vi "Find Parameter by Name.vi"(8 "error in":errorcluster, 10 "parameter name":string, 11 "label ref":T1 format="%.0x") -> (0 "error out":errorcluster, 2 "parameter ref":T1 format="%.0x", 3 "label ref out":T1 format="%.0x", 4 "found?":bool)   [LabVIEW 2024, in "AIM ARINC 429 Scripting.lvlib"]
doc: "Within the specified <b>label ref</b>, this VI searches for a parameter with matching <b>parameter name</b>. If a match is found, returns the matching <b>parameter</b> reference. If no match is found, the returned reference is invalid and <b>found?</b> equals False."
uses:
  AIM ARINC 429 Scripting.lvlib
  <vilib>/NI VeriStand/Custom Device API/Custom Device Item Ref.ctl
  <vilib>/NI VeriStand/Custom Device Tools/Custom Device Utility Library/NI VeriStand - Search for Item by Name.vi
  <vilib>/NI VeriStand/Custom Device Tools/Custom Device Utility Library/Custom Device Utility Library.lvlib
  <vilib>/NI VeriStand/Custom Device API/Custom Device API.lvlib
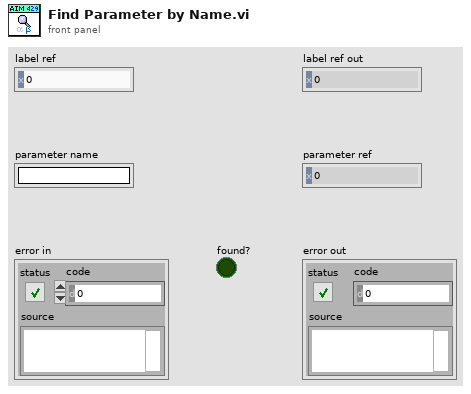
[diagram p1: front panel]
types:
  T1 = typedef "Custom Device API.lvlib/Custom Device Item Ref.ctl" = u64
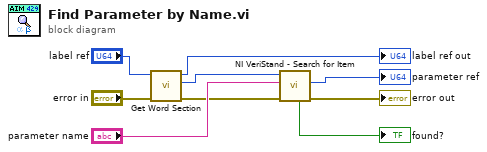
[diagram p0: block diagram]
diagram:
  n1 = call "Get Word Section.vi"("error in"="error in", "label ref"="label ref") -> ("error out"=w1:errorcluster, "word ref"=w4:T1, "label ref out"=→"label ref out":T1)  [unwired: 7 in]
  n2 = call-poly <vilib>:"NI VeriStand - Search for Item.vi"("error in"=w1, "Item Name"="parameter name", "Section Ref in"=w4) -> ("error out"=→"error out":errorcluster, "Item Ref"=→"parameter ref":T1, "Found"=→"found?":bool)  [unwired: 5 in, 1 out]
